vi "LVObject to JSON - 200 Elements - Produces Pretty Output.vi"() -> ()   [LabVIEW 2017, in "Tests.lvlib" / "Pretty Print.lvlib"]
uses:
  Pretty Print.lvlib
  Flatten To JSON Object/Flatten To JSON Object.lvclass
  Strings/Strings.lvclass
  <vilib>/addons/_JKI Toolkits/Caraya/classes/Assert/Assert Equal Value_Variant.vi
  <vilib>/addons/_JKI Toolkits/Caraya/classes/Test/Test.lvclass
  <vilib>/addons/_JKI Toolkits/Caraya/classes/Assert/Assert.lvclass
panel:
  out "error out":errorcluster
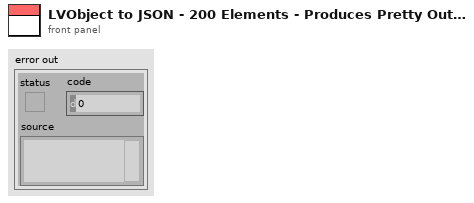
[diagram p1: front panel]
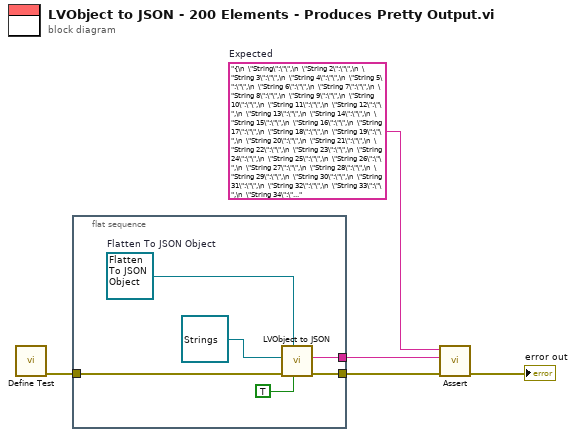
[diagram p0: block diagram]
diagram:
  w1 = "{\n  \"String\":\"\",\n  \"String 2\":\"\",\n  \"String 3\":\"\",\n  \"String 4\":\"\",\n  \"String 5\":\"\",\n  \"String 6\":\"\",\n  \"String 7\":\"\",\n  \"String 8\":\"\",\n  \"String 9\":\"\",\n  \"String 10\":\"\",\n  \"String 11\":\"\",\n  \"String 12\":\"\",\n  \"String 13\":\"\",\n  \"String 14\":\"\",\n  \"String 15\":\"\",\n  \"String 16\":\"\",\n  \"String 17\":\"\",\n  \"String 18\":\"\",\n  \"String 19\":\"\",\n  \"String 20\":\"\",\n  \"String 21\":\"\",\n  \"String 22\":\"\",\n  \"String 23\":\"\",\n  \"String 24\":\"\",\n  \"String 25\":\"\",\n  \"String 26\":\"\",\n  \"String 27\":\"\",\n  \"String 28\":\"\",\n  \"String 29\":\"\",\n  \"String 30\":\"\",\n  \"String 31\":\"\",\n  \"String 32\":\"\",\n  \"String 33\":\"\",\n  \"String 34\":\"\",\n  \"String 35\":\"\",\n  \"String 36\":\"\",\n  \"String 37\":\"\",\n  \"String 38\":\"\",\n  \"String 39\":\"\",\n  \"String 40\":\"\",\n  \"String 41\":\"\",\n  \"String 42\":\"\",\n  \"String 43\":\"\",\n  \"String 44\":\"\",\n  \"String 45\":\"\",\n  \"String 46\":\"\",\n  \"String 47\":\"\",\n  \"String 48\":\"\",\n  \"String 49\":\"\",\n  \"String 50\":\"\",\n  \"String 51\":\"\",\n  \"String 52\":\"\",\n  \"String 53\":\"\",\n  \"String 54\":\"\",\n  \"String 55\":\"\",\n  \"String 56\":\"\",\n  \"String 57\":\"\",\n  \"String 58\":\"\",\n  \"String 59\":\"\",\n  \"String 60\":\"\",\n  \"String 61\":\"\",\n  \"String 62\":\"\",\n  \"String 63\":\"\",\n  \"String 64\":\"\",\n  \"String 65\":\"\",\n  \"String 66\":\"\",\n  \"String 67\":\"\",\n  \"String 68\":\"\",\n  \"String 69\":\"\",\n  \"String 70\":\"\",\n  \"String 71\":\"\",\n  \"String 72\":\"\",\n  \"String 73\":\"\",\n  \"String 74\":\"\",\n  \"String 75\":\"\",\n  \"String 76\":\"\",\n  \"String 77\":\"\",\n  \"String 78\":\"\",\n  \"String 79\":\"\",\n  \"String 80\":\"\",\n  \"String 81\":\"\",\n  \"String 82\":\"\",\n  \"String 83\":\"\",\n  \"String 84\":\"\",\n  \"String 85\":\"\",\n  \"String 86\":\"\",\n  \"String 87\":\"\",\n  \"String 88\":\"\",\n  \"String 89\":\"\",\n  \"String 90\":\"\",\n  \"String 91\":\"\",\n  \"String 92\":\"\",\n  \"String 93\":\"\",\n  \"String 94\":\"\",\n  \"String 95\":\"\",\n  \"String 96\":\"\",\n  \"String 97\":\"\",\n  \"String 98\":\"\",\n  \"String 99\":\"\",\n  \"String 100\":\"\",\n  \"String 101\":\"\",\n  \"String 102\":\"\",\n  \"String 103\":\"\",\n  \"String 104\":\"\",\n  \"String 105\":\"\",\n  \"String 106\":\"\",\n  \"String 107\":\"\",\n  \"String 108\":\"\",\n  \"String 109\":\"\",\n  \"String 110\":\"\",\n  \"String 111\":\"\",\n  \"String 112\":\"\",\n  \"String 113\":\"\",\n  \"String 114\":\"\",\n  \"String 115\":\"\",\n  \"String 116\":\"\",\n  \"String 117\":\"\",\n  \"String 118\":\"\",\n  \"String 119\":\"\",\n  \"String 120\":\"\",\n  \"String 121\":\"\",\n  \"String 122\":\"\",\n  \"String 123\":\"\",\n  \"String 124\":\"\",\n  \"String 125\":\"\",\n  \"String 126\":\"\",\n  \"String 127\":\"\",\n  \"String 128\":\"\",\n  \"String 129\":\"\",\n  \"String 130\":\"\",\n  \"String 131\":\"\",\n  \"String 132\":\"\",\n  \"String 133\":\"\",\n  \"String 134\":\"\",\n  \"String 135\":\"\",\n  \"String 136\":\"\",\n  \"String 137\":\"\",\n  \"String 138\":\"\",\n  \"String 139\":\"\",\n  \"String 140\":\"\",\n  \"String 141\":\"\",\n  \"String 142\":\"\",\n  \"String 143\":\"\",\n  \"String 144\":\"\",\n  \"String 145\":\"\",\n  \"String 146\":\"\",\n  \"String 147\":\"\",\n  \"String 148\":\"\",\n  \"String 149\":\"\",\n  \"String 150\":\"\",\n  \"String 151\":\"\",\n  \"String 152\":\"\",\n  \"String 153\":\"\",\n  \"String 154\":\"\",\n  \"String 155\":\"\",\n  \"String 156\":\"\",\n  \"String 157\":\"\",\n  \"String 158\":\"\",\n  \"String 159\":\"\",\n  \"String 160\":\"\",\n  \"String 161\":\"\",\n  \"String 162\":\"\",\n  \"String 163\":\"\",\n  \"String 164\":\"\",\n  \"String 165\":\"\",\n  \"String 166\":\"\",\n  \"String 167\":\"\",\n  \"String 168\":\"\",\n  \"String 169\":\"\",\n  \"String 170\":\"\",\n  \"String 171\":\"\",\n  \"String 172\":\"\",\n  \"String 173\":\"\",\n  \"String 174\":\"\",\n  \"String 175\":\"\",\n  \"String 176\":\"\",\n  \"String 177\":\"\",\n  \"String 178\":\"\",\n  \"String 179\":\"\",\n  \"String 180\":\"\",\n  \"String 181\":\"\",\n  \"String 182\":\"\",\n  \"String 183\":\"\",\n  \"String 184\":\"\",\n  \"String 185\":\"\",\n  \"String 186\":\"\",\n  \"String 187\":\"\",\n  \"String 188\":\"\",\n  \"String 189\":\"\",\n  \"String 190\":\"\",\n  \"String 191\":\"\",\n  \"String 192\":\"\",\n  \"String 193\":\"\",\n  \"String 194\":\"\",\n  \"String 195\":\"\",\n  \"String 196\":\"\",\n  \"String 197\":\"\",\n  \"String 198\":\"\",\n  \"String 199\":\"\",\n  \"String 200\":\"\"\n}"  # Expected
  n1 = call <vilib>:"Define Test.vi"() -> ("error out"=w4:errorcluster)  [unwired: 11 in]
  n2 = flat-sequence {
    tunnel: w4 -> [w8]
    tunnel: [w10] -> w3
    tunnel: [w9] -> w2
    frame #0 {
      w11 = refnum<class "Flatten To JSON Object.lvclass"> refnum  # Flatten To JSON Object
      n3 = call-dynamic "LVObject to JSON.vi"("Pretty Print?"=TRUE, "LVClass Serializer"=w11, "error in (no error)"=w8, "Object"=refnum<class "Strings.lvclass"> refnum ("Tests.lvlib:Strings.lvclass")) -> ("error out"=w10:errorcluster, "<JSON>Object"=w9:string)  [unwired: 6 in]
    }
  }
  n4 = call-poly <vilib>:"Assert.vi"("error in (no error)"=w3, "Y"=w2, "X"=w1) -> ("error out"=→"error out":errorcluster)  [unwired: 8 in]
